vi "Excel Veri Okuma Deneme.vi"() -> ()   [LabVIEW 2014]
panel:
  out "Read Values Array":dbl[][](array[numeric])
  in  "File Name":string="denemem"
  out "error out":errorcluster
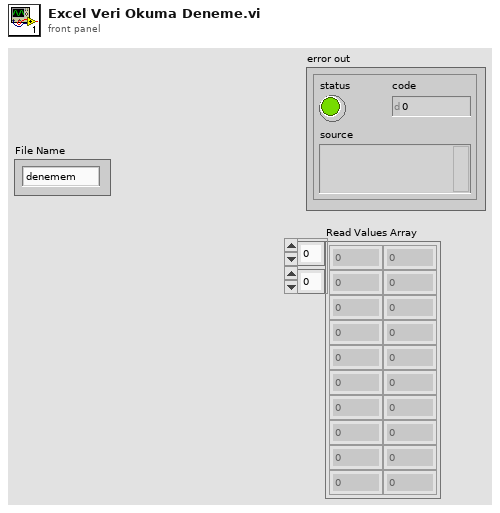
[diagram p1: front panel]
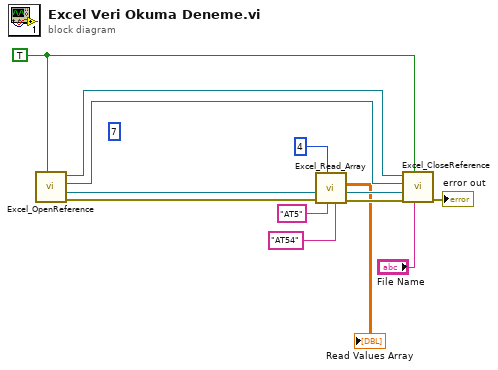
[diagram p0: block diagram]
diagram:
  (unwired) 7
  w9 = TRUE ("File Visible ?")
  n1 = call "Excel_OpenReference.vi"("File Visible ?"=w9) -> ("error out"=w6:errorcluster, "Sheets Reference Out"=w5:refnum<k7>, "Workbook Reference Out"=w10:refnum<k7>, "Excel Application Reference Out"=w11:refnum<k7>)  [unwired: 7 in]
  n2 = call "Excel_Read_Array.vi"("Cell Range 2"="AT54", "Cell Range 1"="AT5" ("Cell to Read"), "Worksheet Number"=4, "error in (no error)"=w6, "Sheets Reference In"=w5) -> ("error out"=w13:errorcluster, "Sheets Reference Out"=w12:refnum<k7>, "Read Values Array"=→"Read Values Array":dbl[][])  [unwired: 4 in]
  n3 = call "Excel_CloseReference.vi"("File Name"="File Name", "Keep Excel Open ?"=w9, "error in (no error)"=w13, "Sheets Reference In"=w12, "Workbook Reference In"=w10, "Excel Application Reference In"=w11) -> ("error out"=→"error out":errorcluster)  [unwired: 5 in]
